vi "ErrCheck_Valid Instruction Name.vi"(8 "Error In":errorcluster, 11 "Macro Command String IN":string="LOOP.Start\t(loop.iterations,3.000);") -> (0 "Error Out":errorcluster, 2 "Generic Instruction?":bool, 3 "Invalid Instruction name?":bool)   [LabVIEW 2012]
doc: "SciScan 1.2 160622"
uses:
  <vilib>/Utility/error.llb/whitespace.ctl
  MacroRules_FGV_Commands.ctl
panel:
  out "Instruction":string
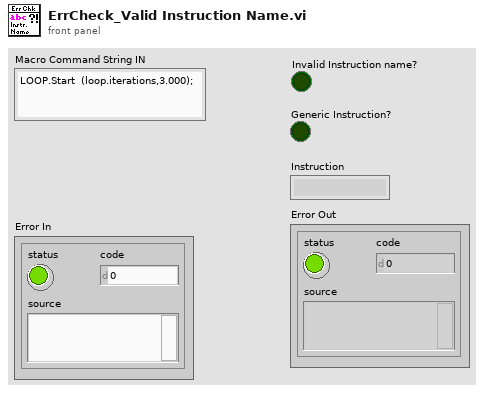
[diagram p1: front panel]
types:
  T1 = typedef "MacroRules_FGV_Commands.ctl" = enum16{"Read File", "Get All", "Get Param and Flags"}
  T2 = typedef "whitespace.ctl" = u16
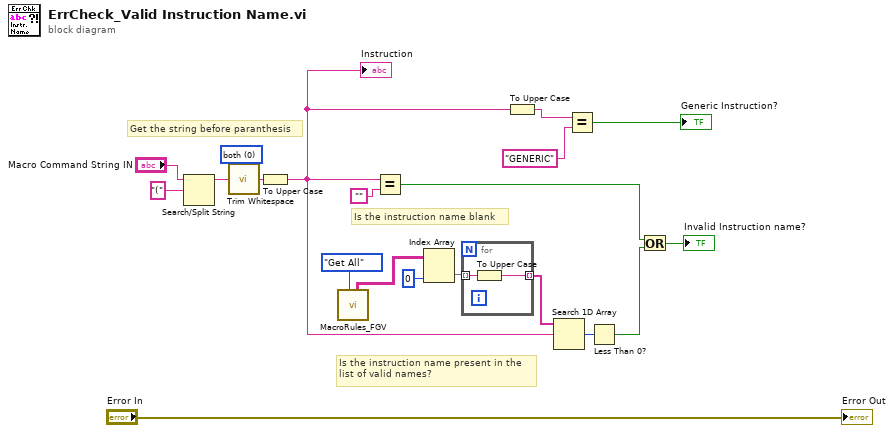
[diagram p0: block diagram]
diagram:
  w18 = T2 0 items=["both", "start of string", "end of string"] ("location (both)")
  # "Is the instruction name present in the\nlist of valid names?"
  # "Is the instruction name blank"
  # "Get the string before paranthesis"
  n1 = Search/Split String(string="Macro Command String IN", search string/char (-)="(") -> (substring before match=w12:string)  [unwired: 1 in, 2 out]
  n2 = call <vilib>:"Trim Whitespace.vi"("string"=w12, "location (both)"=w18) -> ("trimmed string"=w3:string)
  n3 = To Upper Case(1:w3) -> (0:w2:string)
  "Instruction" <- w2
  n4 = call "MacroRules_FGV.vi"("MacroRules_FGV_Commands"=MacroRules_FGV_Commands."Get All") -> ("ParametersTable"=w13:string[][])  [unwired: 6 in, 4 out]
  n5 = Equal?(x=w2, y="") -> (x = y?=w10:bool)
  n6 = Index Array(array=w13, index (col)=0 ("disabled index (col)")) -> (element=w4:string[])  [unwired: 1 in]
  n7 = for {
    tunnel: w4 -> [w22] mode=indexing
    tunnel: [w21] -> w1 mode=indexing
    n8 = To Upper Case(1:w22) -> (0:w21:string)
  }
  n9 = To Upper Case(1:w2) -> (0:w6:string)
  n10 = Search 1D Array(1D array=w1, element=w2) -> (index of element=w14:i32)  [unwired: 1 in]
  n11 = Equal?(x=w6, y="GENERIC" ("search string/char (-)")) -> (x = y?=→"Generic Instruction?":bool)
  n12 = Less Than 0?(x=w14) -> (x < 0?=w9:bool)
  n13 = Or(x=w10, y=w9) -> (x .or. y?=→"Invalid Instruction name?":bool)
  "Error Out" <- "Error In"
